vi "Pump_API_Application_Test.vi"() -> ()   [LabVIEW 2021]
uses:
  labbCAN_Bus_API/SiUnitPrefix.ctl
  labbCAN_Pump_API/VolumeUnits.ctl
  labbCAN_Bus_API/TimeUnits.ctl
  labbCAN_Bus_API/labbCAN_Bus_API.lvlib
  labbCAN_Pump_API/labbCAN_Pump_API.lvlib
  labbCAN_Valve_API/labbCAN_Valve_API.lvlib
panel:
  out "error out":errorcluster caption="Fehler (Ausgang)"
  in  "Stop Dosage":bool
  in  "Empty":bool
  in  "Refill":bool
  in  "Generate Flow":bool
  in  "SetSyringeLevel":bool
  in  "Flow rate":dbl caption="Flow rate (ml/min)" min=-28425000.0 max=28425331.391610276 step=1.0 format="%.6g"
  in  "Target Syringe Level":dbl caption="Target syringe level (ml)" min=0.0 max=6333.029896332054 step=1.0 format="%.6g"
  out "Actual flow rate":dbl caption="Actual flow rate (ml/min)"
  out "Syringe":dbl(slide) caption="Actual syringe level (ml)" max=6333.029896332054 scale=0.0..6333.029896332054 scale format="%.3g"
  out "Is pumping":bool
  out "Valve position":i32
  out "Valve positions":i32
  out "Has valve":bool
  in  "Calibrate":bool
  out "Pump handle":i64
  out "Application Directory":path caption="Applikationsverzeichnis"
  out "Config Path":string
  out "Connected":bool
  in  "Connect":bool
  out "Run":bool
  # "Target values"
  # "Commands"
  # "Actual values"
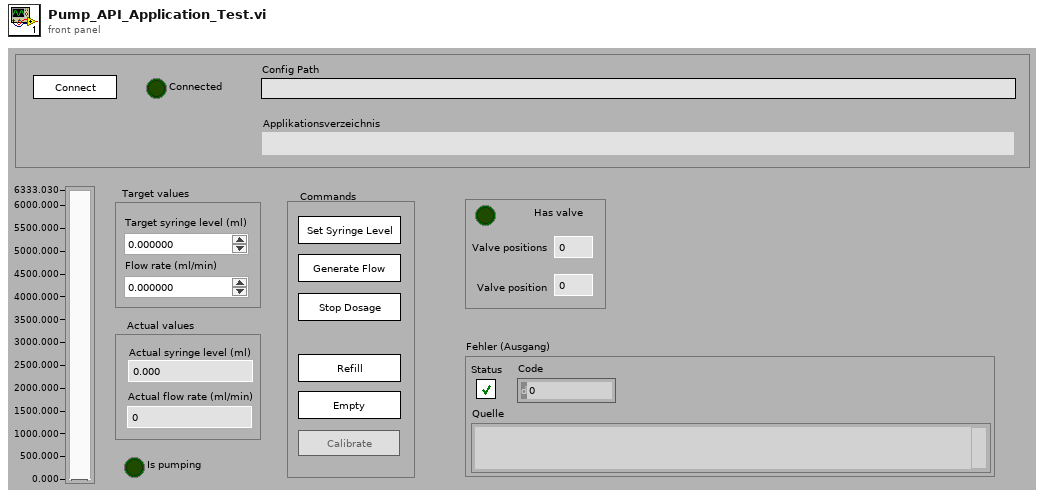
[diagram p1: front panel]
types:
  T1 = enum8{"Enabled", "Disabled", "Disabled and Grayed Out"}
  T2 = typedef "labbCAN_Bus_API.lvlib/TimeUnits.ctl" = i32
  T3 = typedef "labbCAN_Pump_API.lvlib/VolumeUnits.ctl" = i32
  T4 = typedef "labbCAN_Bus_API.lvlib/SiUnitPrefix.ctl" = i32
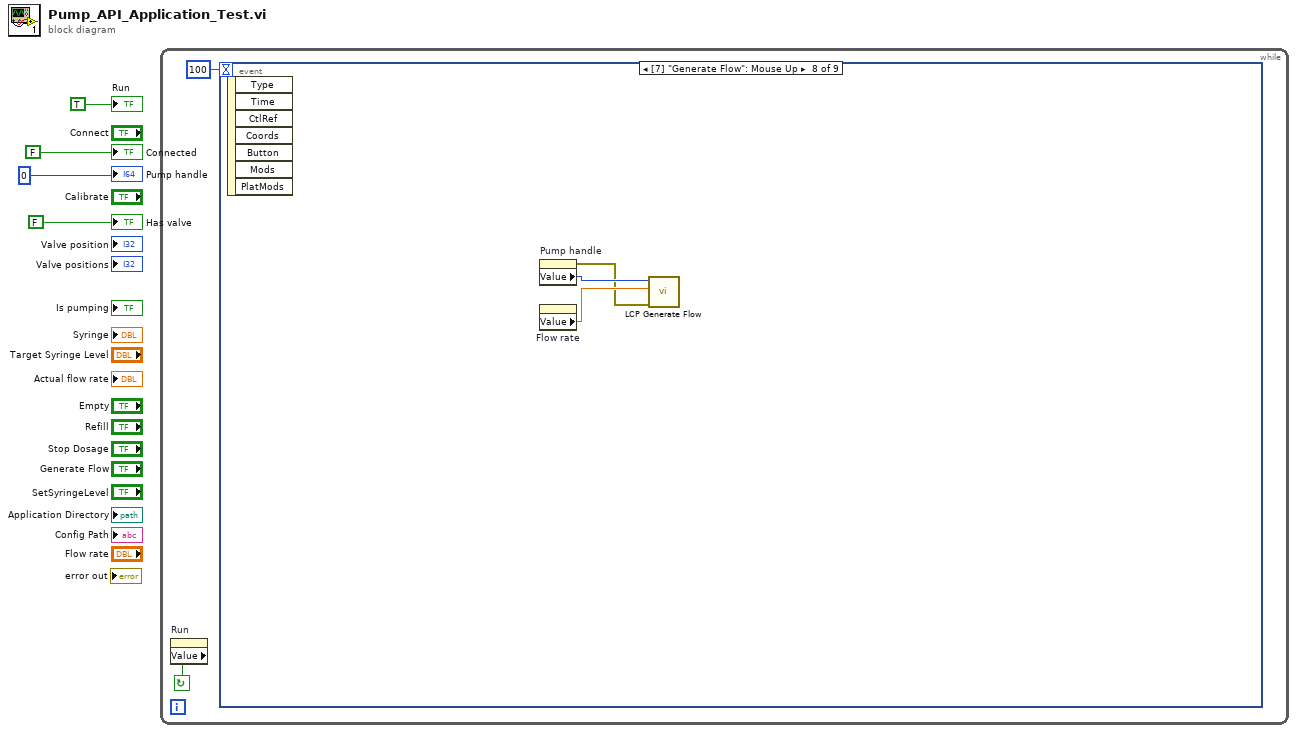
[diagram p0: block diagram]
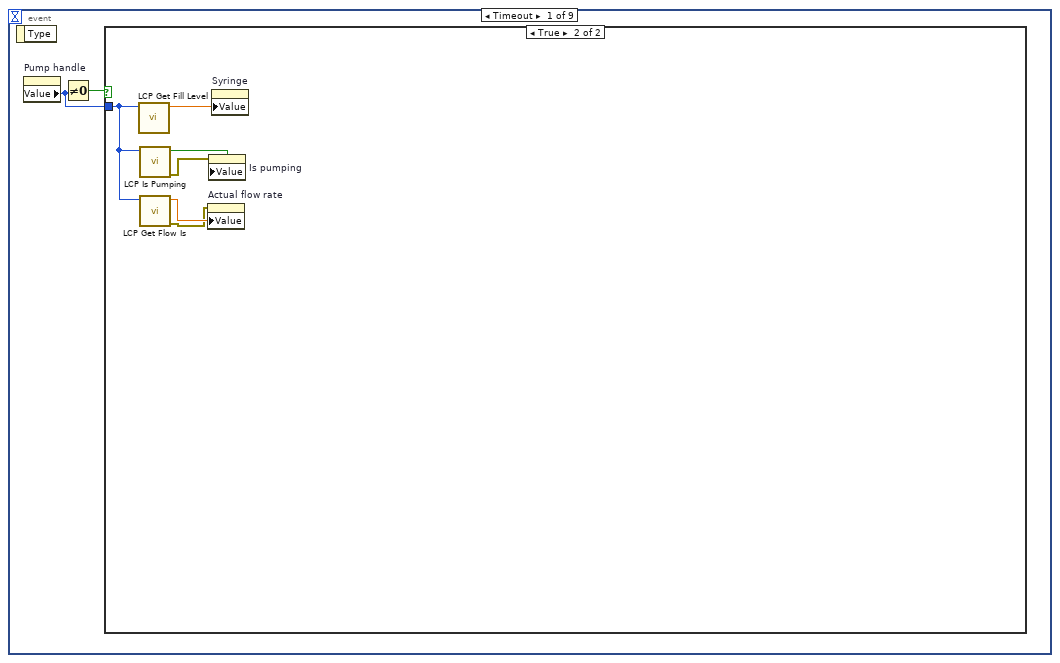
[diagram p2: hidden frame]
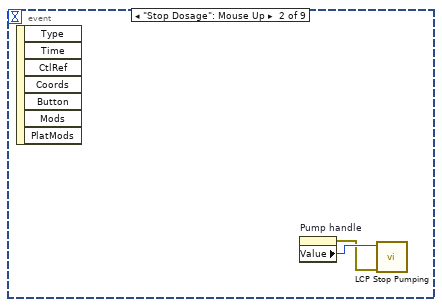
[diagram p4: hidden frame]
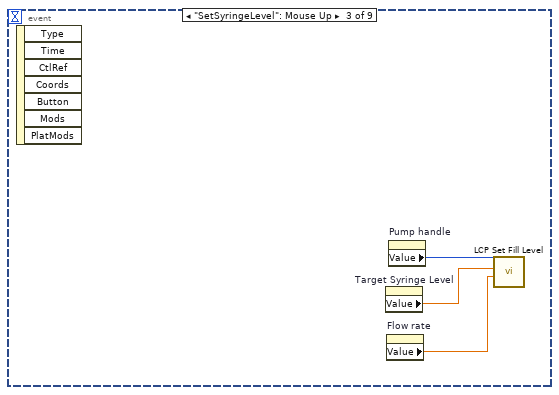
[diagram p5: hidden frame]
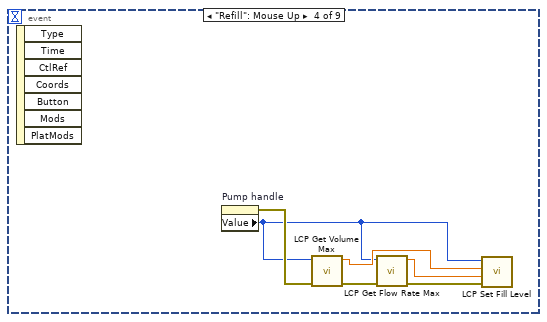
[diagram p6: hidden frame]
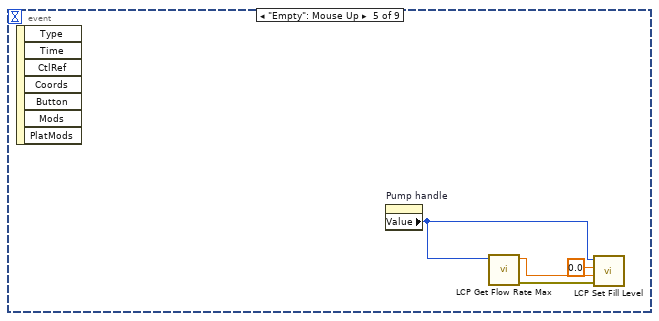
[diagram p7: hidden frame]
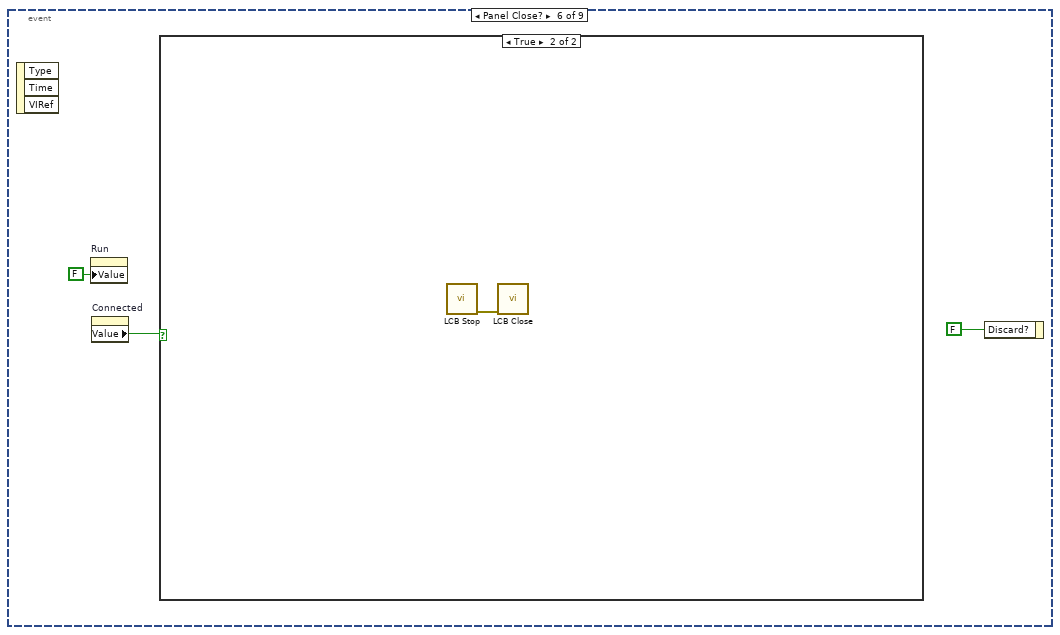
[diagram p8: hidden frame]
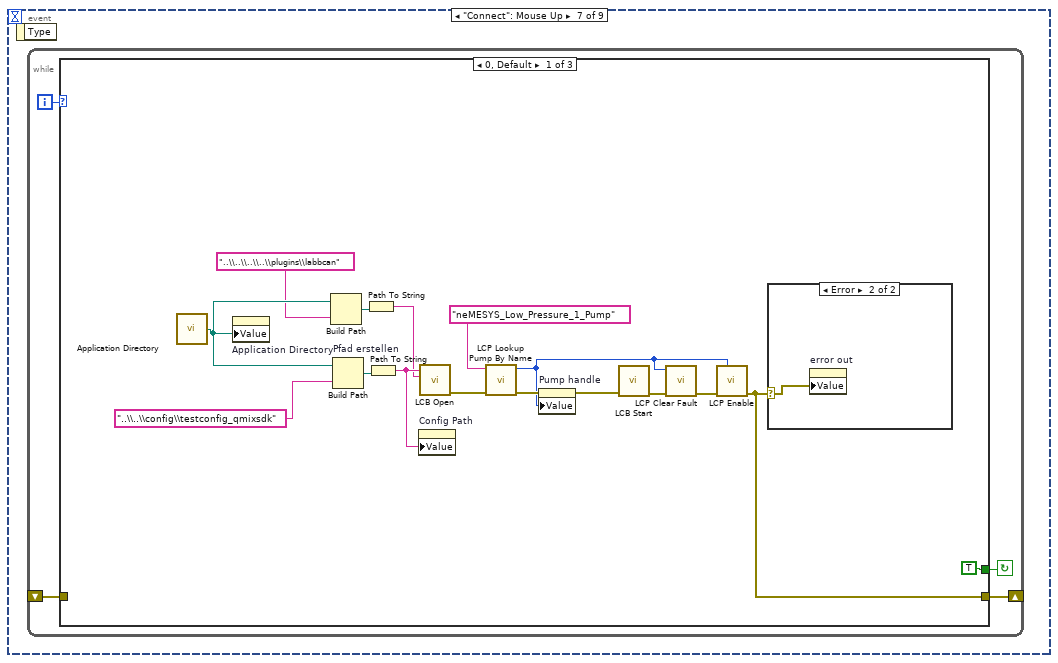
[diagram p10: hidden frame]
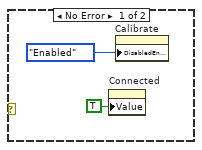
[diagram p11: hidden frame]
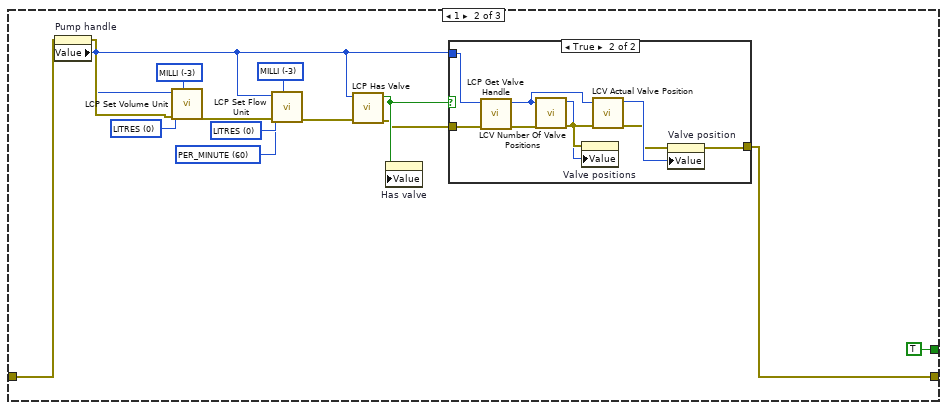
[diagram p12: hidden frame]
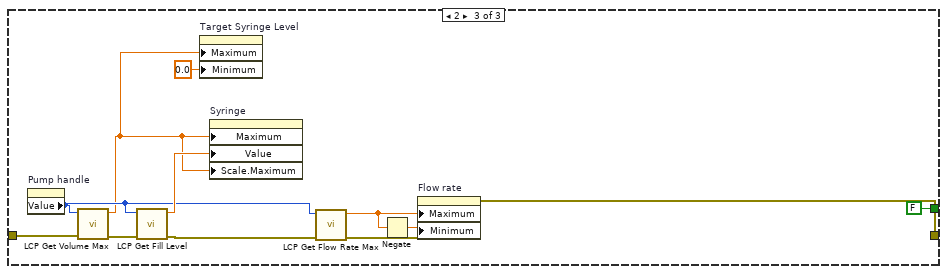
[diagram p14: hidden frame]
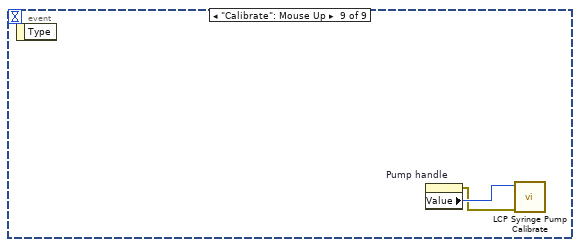
[diagram p15: hidden frame]
diagram:
  n1 = while {
    stop <- w6 continue-if-true
    n2 = property on="Run" class="Bool (strict)"() -> ("Value"=w6:bool)  [unwired: 2 in, 2 out]
    n3 = event shown="[7] \"Generate Flow\": Mouse Up" {
      selector: _ -> [_ _ _ _ _ _ _ _ _]
      dyn-events: _ -> [_ _ _ _ _ _ _ _ _]
      timeout: 100 -> [_ _ _ _ _ _ _ _ _]
      event Timeout {
        n4 = event-data() -> ()  [unwired: 1 in, 1 out]
        n5 = property on="Pump handle" class="DigNum (strict)"() -> ("Value"=w7:i64)  [unwired: 2 in, 2 out]
        n6 = Not Equal To 0?(x=w7) -> (x != 0?=w8:bool)
        n7 = case shown="True" w8 {
          tunnel: w7 -> [_ w11]
          frame False {
          }
          frame True {
            n8 = call "LCP Get Fill Level.vi"("Pump Handle"=w11) -> ("Fill Level"=w12:dbl)  [unwired: 9 in, 1 out]
            n9 = call "LCP Is Pumping.vi"("Pump Handle"=w11) -> ("error out"=w14:errorcluster, "Is pumping"=w13:bool)  [unwired: 9 in]
            n10 = call "LCP Get Flow Is.vi"("Pump Handle"=w11) -> ("error out"=w9:errorcluster, "Actual Flow Rate"=w10:dbl)  [unwired: 9 in]
            n11 = property on="Actual flow rate" class="DigNum (strict)"(error in=w9, "Value"=w10) -> ()  [unwired: 1 in, 2 out]
            n12 = property on="Is pumping" class="Bool (strict)"(error in=w14, "Value"=w13) -> ()  [unwired: 1 in, 2 out]
            n13 = property on="Syringe" class="Slide (strict)"("Value"=w12) -> ()  [unwired: 2 in, 2 out]
          }
        }
      }
      event "Stop Dosage": Mouse Up {
        n14 = event-data() -> ()  [unwired: 1 in, 7 out]
        n15 = property on="Pump handle" class="DigNum (strict)"() -> (error out=w15:errorcluster, "Value"=w16:i64)  [unwired: 2 in, 1 out]
        n16 = call "LCP Stop Pumping.vi"("error in (no error)"=w15, "Pump Handle"=w16) -> ()  [unwired: 9 in, 1 out]
      }
      event "SetSyringeLevel": Mouse Up {
        n17 = event-data() -> ()  [unwired: 1 in, 7 out]
        n18 = property on="Target Syringe Level" class="DigNum (strict)"() -> ("Value"=w18:dbl)  [unwired: 2 in, 2 out]
        n19 = property on="Flow rate" class="DigNum (strict)"() -> ("Value"=w17:dbl)  [unwired: 2 in, 2 out]
        n20 = property on="Pump handle" class="DigNum (strict)"() -> ("Value"=w19:i64)  [unwired: 2 in, 2 out]
        n21 = call "LCP Set Fill Level.vi"("Flow"=w17, "Level"=w18, "Pump Handle"=w19) -> ()  [unwired: 8 in, 1 out]
      }
      event "Refill": Mouse Up {
        n22 = event-data() -> ()  [unwired: 1 in, 7 out]
        n23 = property on="Pump handle" class="DigNum (strict)"() -> (error out=w25:errorcluster, "Value"=w20:i64)  [unwired: 2 in, 1 out]
        n24 = call "LCP Get Volume Max.vi"("error in (no error)"=w25, "Pump Handle"=w20) -> ("error out"=w24:errorcluster, "Maximum Volume"=w21:dbl)  [unwired: 8 in]
        n25 = call "LCP Get Flow Rate Max.vi"("error in (no error)"=w24, "Pump Handle"=w20) -> ("error out"=w23:errorcluster, "Maximum Flow Rate"=w22:dbl)  [unwired: 8 in]
        n26 = call "LCP Set Fill Level.vi"("error in (no error)"=w23, "Flow"=w22, "Level"=w21, "Pump Handle"=w20) -> ()  [unwired: 7 in, 1 out]
      }
      event "Empty": Mouse Up {
        n27 = event-data() -> ()  [unwired: 1 in, 7 out]
        n28 = property on="Pump handle" class="DigNum (strict)"() -> ("Value"=w26:i64)  [unwired: 2 in, 2 out]
        n29 = call "LCP Get Flow Rate Max.vi"("Pump Handle"=w26) -> ("error out"=w29:errorcluster, "Maximum Flow Rate"=w28:dbl)  [unwired: 9 in]
        n30 = call "LCP Set Fill Level.vi"("error in (no error)"=w29, "Flow"=w28, "Level"=0.0, "Pump Handle"=w26) -> ()  [unwired: 7 in, 1 out]
      }
      event Panel Close? {
        n31 = event-data() -> ()  [unwired: 1 in, 3 out]
        n32 = property on="Run" class="Bool (strict)"("Value"=FALSE ("Run")) -> ()  [unwired: 2 in, 2 out]
        n33 = property on="Connected" class="Bool (strict)"() -> ("Value"=w30:bool)  [unwired: 2 in, 2 out]
        n34 = case shown="True" w30 {
          frame False {
          }
          frame True {
            n35 = call "LCB Stop.vi"() -> ("error out"=w33:errorcluster)  [unwired: 11 in]
            n36 = call "LCB Close.vi"("error in (no error)"=w33) -> ()  [unwired: 10 in, 1 out]
          }
        }
        n37 = event-data("Discard?"=FALSE ("Verwerfen?")) -> ()  [unwired: 1 in, 1 out]
      }
      event "Connect": Mouse Up {
        n38 = event-data() -> ()  [unwired: 1 in, 1 out]
        n39 = while {
          shift-right: [w35] -> _
          shift-left: _ -> [w34]
          i -> [w37]
          stop <- w36 continue-if-true
          n40 = case shown="0, Default" w37 {
            tunnel: [TRUE TRUE FALSE] -> w36
            tunnel: [w40 w58 w83] -> w35
            tunnel: w34 -> [_ w61 w91]
            frame 0, Default {
              n41 = call <vilib>:"Application Directory.vi"() -> ("Application Directory"=w52:path)
              n42 = property on="Application Directory" class="Path"("Value"=w52) -> ()  [unwired: 2 in, 2 out]
              n43 = Build Path(base path=w52, name or relative path="..\\..\\..\\..\\plugins\\labbcan" ("Name oder relativer Pfad")) -> (appended path=w49:path)
              n44 = Build Path "Pfad erstellen"(base path=w52, name or relative path="..\\..\\config\\testconfig_qmixsdk" ("Name oder relativer Pfad")) -> (appended path=w47:path)
              n45 = Path To String(path=w49) -> (string=w48:string)
              n46 = Path To String(path=w47) -> (string=w53:string)
              n47 = property on="Config Path" class="Str"("Value"=w53) -> ()  [unwired: 2 in, 2 out]
              n48 = call "LCB Open.vi"("PluginSearchPath"=w48, "Device Configuration Path"=w53) -> ("error out"=w51:errorcluster)  [unwired: 9 in]
              n49 = call "LCP Lookup Pump By Name.vi"("error in (no error)"=w51, "Pump Name"="neMESYS_Low_Pressure_1_Pump" ("pAxisName")) -> ("error out"=w45:errorcluster, "Pump handle"=w42:i64)  [unwired: 8 in]
              n50 = property on="Pump handle" class="DigNum (strict)"(error in=w45, "Value"=w42) -> (error out=w46:errorcluster)  [unwired: 1 in, 1 out]
              n51 = call "LCB Start.vi"("error in (no error)"=w46) -> ("error out"=w44:errorcluster)  [unwired: 10 in]
              n52 = call "LCP Clear Fault.vi"("error in (no error)"=w44, "Pump Handle"=w42) -> ("error out"=w43:errorcluster)  [unwired: 9 in]
              n53 = call "LCP Enable.vi"("error in (no error)"=w43, "Pump Handle"=w42) -> ("error out"=w40:errorcluster)  [unwired: 9 in]
              n54 = case shown="Error" w40 {
                selector: w40 -> [_ w56]
                frame No Error {
                  n55 = property on="Connected" class="Bool (strict)"("Value"=TRUE ("Connected")) -> ()  [unwired: 2 in, 2 out]
                  n56 = property on="Calibrate" class="Bool (strict)"("DisabledEnum"=T1."Enabled" ("Deaktiviert")) -> ()  [unwired: 2 in, 2 out]
                }
                frame Error {
                  n57 = property on="error out" class="Clust (strict)"("Value"=w56) -> ()  [unwired: 2 in, 2 out]
                }
              }
            }
            frame 1 {
              w64 = T2 60 items=["PER_SECOND"=1, "PER_MINUTE"=60, "PER_HOUR"=3600] ("TimeUnit")
              w65 = T3 0 items=["LITRES"] ("VolumeUnit")
              w66 = T3 0 items=["LITRES"] ("Volume Unit")
              w67 = T4 -3 items=["UNIT"=0, "DECI"=-1, "CENTI"=-2, "MILLI"=-3, "MICRO"=-6] ("Prefix")
              w69 = T4 -3 items=["UNIT"=0, "DECI"=-1, "CENTI"=-2, "MILLI"=-3, "MICRO"=-6] ("Prefix")
              n58 = property on="Pump handle" class="DigNum (strict)"(error in=w61) -> (error out=w62:errorcluster, "Value"=w57:i64)  [unwired: 1 in, 1 out]
              n59 = call "LCP Set Volume Unit.vi"("Prefix"=w69, "error in (no error)"=w62, "Volume Unit"=w66, "Pump Handle"=w57) -> ("error out"=w68:errorcluster)  [unwired: 7 in]
              n60 = call "LCP Set Flow Unit.vi"("Prefix"=w67, "error in (no error)"=w68, "TimeUnit"=w64, "VolumeUnit"=w65, "Pump Handle"=w57) -> ("error out"=w60:errorcluster)  [unwired: 6 in]
              n61 = call "LCP Has Valve.vi"("error in (no error)"=w60, "Pump Handle"=w57) -> ("error out"=w59:errorcluster, "Has Valve"=w63:bool)  [unwired: 8 in]
              n62 = property on="Has valve" class="Bool (strict)"("Value"=w63) -> ()  [unwired: 2 in, 2 out]
              n63 = case shown="True" w63 {
                tunnel: w59 -> [w71 w80]
                tunnel: [w71 w73] -> w58
                tunnel: w57 -> [_ w72]
                frame False {
                }
                frame True {
                  n64 = call "LCP Get Valve Handle.vi"("error in (no error)"=w80, "Pump Handle"=w72) -> ("error out"=w79:errorcluster, "Valve Handle"=w78:i64)  [unwired: 8 in]
                  n65 = call "LCV Number Of Valve Positions.vi"("error in (no error)"=w79, "Valve Handle"=w78) -> ("error out"=w77:errorcluster, "Valve Position Count"=w76:i32)  [unwired: 8 in]
                  n66 = property on="Valve positions" class="DigNum (strict)"(error in=w77, "Value"=w76) -> ()  [unwired: 1 in, 2 out]
                  n67 = call "LCV Actual Valve Position.vi"("error in (no error)"=w77, "Valve Handle"=w78) -> ("error out"=w74:errorcluster, "Actual valve position"=w75:i32)  [unwired: 8 in]
                  n68 = property on="Valve position" class="DigNum (strict)"(error in=w74, "Value"=w75) -> (error out=w73:errorcluster)  [unwired: 1 in, 1 out]
                }
              }
            }
            frame 2 {
              n69 = property on="Pump handle" class="DigNum (strict)"() -> ("Value"=w87:i64)  [unwired: 2 in, 2 out]
              n70 = call "LCP Get Volume Max.vi"("error in (no error)"=w91, "Pump Handle"=w87) -> ("error out"=w90:errorcluster, "Maximum Volume"=w85:dbl)  [unwired: 8 in]
              n71 = call "LCP Get Fill Level.vi"("error in (no error)"=w90, "Pump Handle"=w87) -> ("error out"=w88:errorcluster, "Fill Level"=w89:dbl)  [unwired: 8 in]
              n72 = property on="Target Syringe Level" class="DigNum (strict)"("Maximum"=w85, "Minimum"=0.0 ("Wertebereich:Minimum")) -> ()  [unwired: 2 in, 2 out]
              n73 = property on="Syringe" class="Slide (strict)"("Maximum"=w85, "Value"=w89, "Scale.Maximum"=w85) -> ()  [unwired: 2 in, 2 out]
              n74 = call "LCP Get Flow Rate Max.vi"("error in (no error)"=w88, "Pump Handle"=w87) -> ("error out"=w86:errorcluster, "Maximum Flow Rate"=w81:dbl)  [unwired: 8 in]
              n75 = Negate(x=w81) -> (-x=w82:dbl)
              n76 = property on="Flow rate" class="DigNum (strict)"(error in=w86, "Maximum"=w81, "Minimum"=w82) -> (error out=w83:errorcluster)  [unwired: 1 in, 1 out]
            }
          }
        }
      }
      event "Generate Flow": Mouse Up {
        n77 = event-data() -> ()  [unwired: 1 in, 7 out]
        n78 = property on="Pump handle" class="DigNum (strict)"() -> (error out=w93:errorcluster, "Value"=w95:i64)  [unwired: 2 in, 1 out]
        n79 = property on="Flow rate" class="DigNum (strict)"() -> ("Value"=w94:dbl)  [unwired: 2 in, 2 out]
        n80 = call "LCP Generate Flow.vi"("error in (no error)"=w93, "Flow Rate"=w94, "Pump Handle"=w95) -> ()  [unwired: 8 in, 1 out]
      }
      event "Calibrate": Mouse Up {
        n81 = event-data() -> ()  [unwired: 1 in, 1 out]
        n82 = property on="Pump handle" class="DigNum (strict)"() -> (error out=w96:errorcluster, "Value"=w97:i64)  [unwired: 2 in, 1 out]
        n83 = call "LCP Syringe Pump Calibrate.vi"("error in (no error)"=w96, "Pump Handle"=w97) -> ()  [unwired: 9 in, 1 out]
      }
    }
  }
  "Run" <- TRUE ("Run")
  "Connected" <- FALSE ("Connected")
  "Pump handle" <- i64 0 ("Pump handle")
  "Has valve" <- FALSE ("Has valve")
